vi "Write Beverage.vi"(8 "error in (no error)":errorcluster, 10 "Beverage.lvlib:Beverage.lvclass":refnum<class "Beverage.lvclass">, 11 "Pick up Item Msg in":refnum<class "Pick up Item Msg.lvclass">) -> (0 "error out":errorcluster, 3 "Pick up Item Msg out":refnum<class "Pick up Item Msg.lvclass">)   [LabVIEW 2023, in "Customer.lvlib" / "Pick up Item Msg.lvclass"]
doc: "Simple accessor method to set the Beverage property of the Pick Up Item message."
uses:
  Pick up Item Msg.lvclass
  Beverages/Beverage/Beverage.lvclass
  Pick up Item Msg.lvclass/Pick up Item Msg.ctl
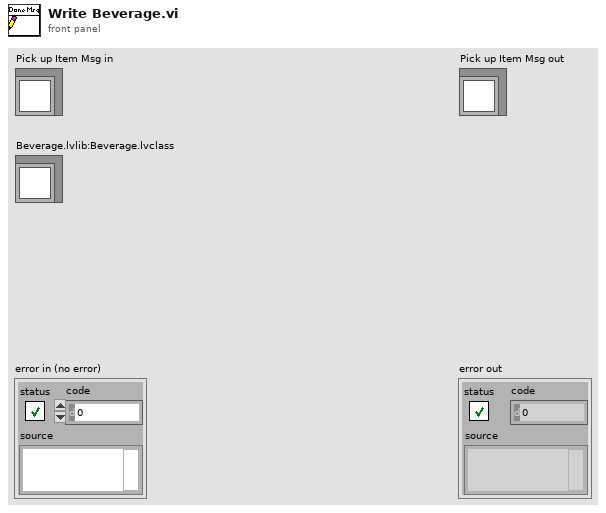
[diagram p1: front panel]
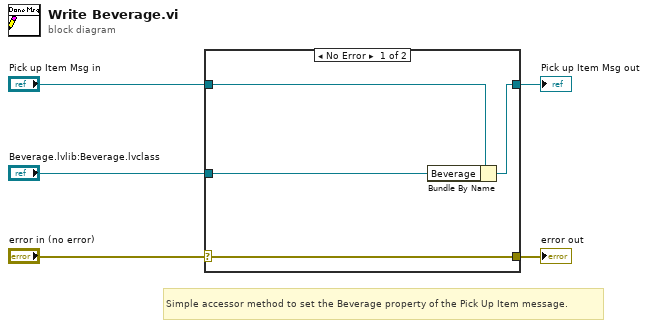
[diagram p0: block diagram]
diagram:
  # "Simple accessor method to set the Beverage property of the Pick Up Item message."
  n1 = case shown="No Error" "error in (no error)" {
    selector: "error in (no error)" -> [w9 w10]
    tunnel: [w9 w10] -> w4
    tunnel: [w7 w11] -> w2
    tunnel: "Pick up Item Msg in" -> [w8 w11]
    tunnel: "Beverage.lvlib:Beverage.lvclass" -> [w6 _]
    frame No Error {
      n2 = Bundle By Name(cluster=w8, "Beverage"=w6) -> (w7:refnum<class "Pick up Item Msg.lvclass">)
    }
    frame Error {
    }
  }
  "error out" <- w4
  "Pick up Item Msg out" <- w2
